vi "PobierzWiadomość.vi"(8 "error in":errorcluster, 9 "Ilość":string, 10 "Konto":T1, 11 "Typ wiadomości":string) -> (0 "error out":errorcluster, 3 "Wiadomość":string)   [LabVIEW 2021]
doc: "Return message in function of the message type\nAnd replace AMOUNT, NAME field in message"
uses:
  Konto.ctl
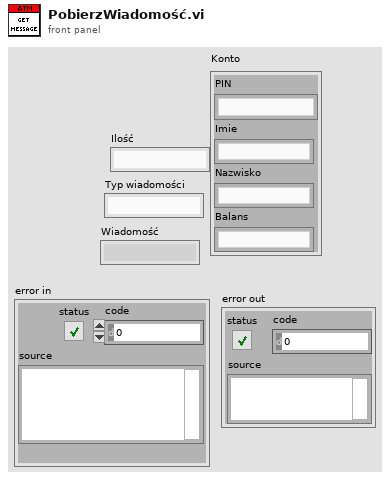
[diagram p1: front panel]
types:
  T1 = typedef "Konto.ctl" = cluster{"PIN":string, "Imie":string, "Nazwisko":string, "Balans":string}
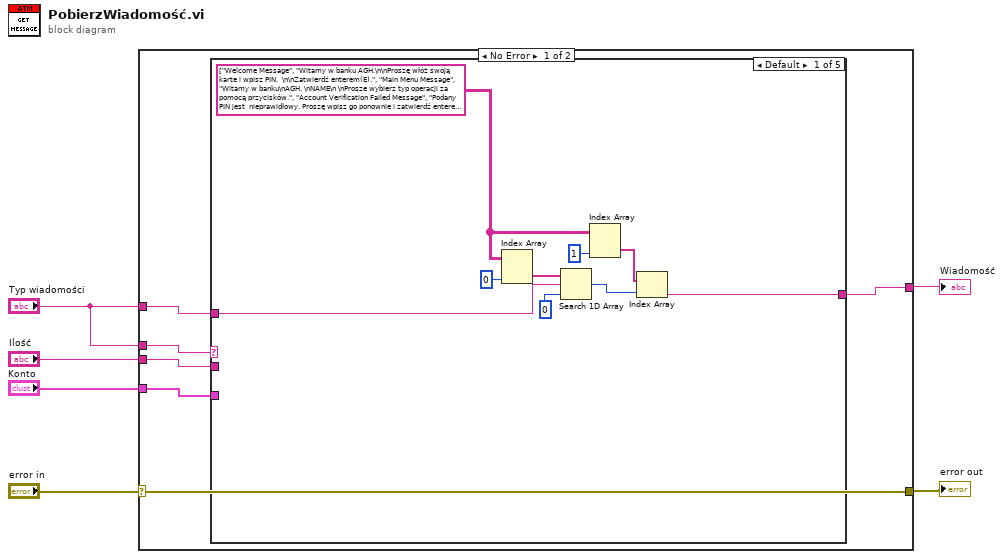
[diagram p0: block diagram]
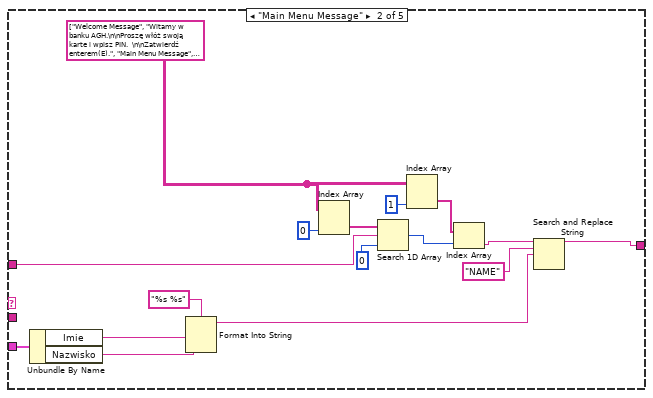
[diagram p2: hidden frame]
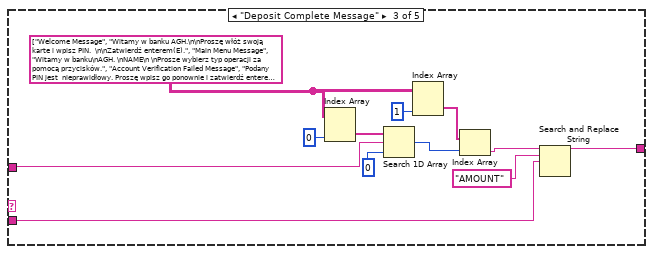
[diagram p3: hidden frame]
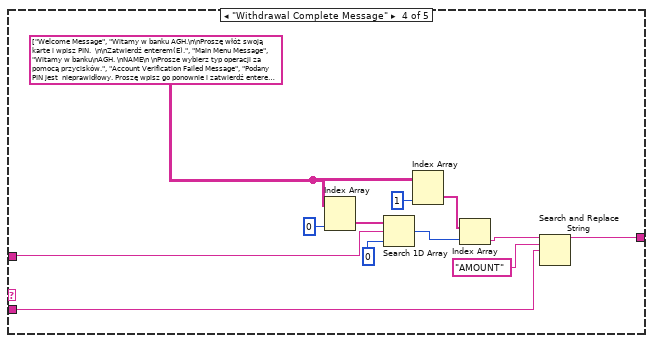
[diagram p4: hidden frame]
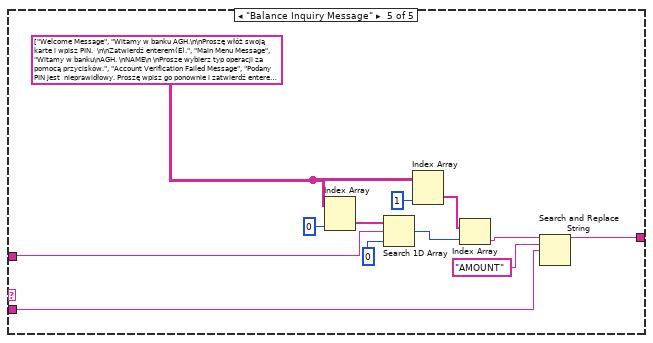
[diagram p5: hidden frame]
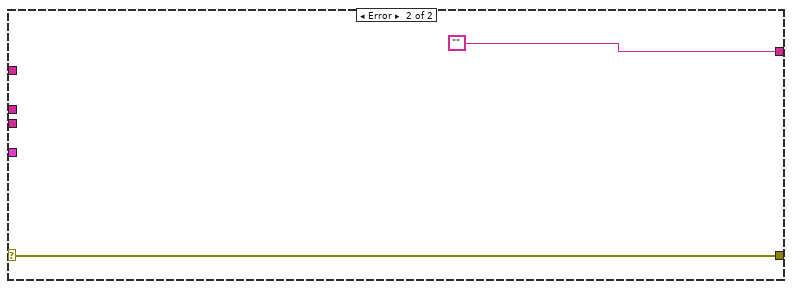
[diagram p6: hidden frame]
diagram:
  n1 = case shown="No Error" "error in" {
    selector: "error in" -> [w10 w75]
    tunnel: "Typ wiadomości" -> [w12 _]
    tunnel: [w11 ""] -> w6
    tunnel: [w10 w75] -> w4
    tunnel: "Typ wiadomości" -> [w9 _]
    tunnel: "Konto" -> [w8 _]
    tunnel: "Ilość" -> [w7 _]
    frame No Error {
      n2 = case shown="Default" w9 {
        tunnel: w12 -> [w14 w31 w40 w52 w64]
        tunnel: [w15 w23 w39 w51 w63] -> w11
        tunnel: w8 -> [_ w29 _ _ _]
        tunnel: w7 -> [_ _ w38 w50 w62]
        frame Default {
          w13 = string[][] [["Welcome Message", "Witamy w banku AGH.\n\nProszę włóż swoją karte i wpisz PIN.  \n\nZatwierdź enterem(E)."], ["Main Menu Message", "Witamy w banku\nAGH. \nNAME\n \nProsze wybierz typ operacji za pomocą przycisków."], ["Account Verification Failed Message", "Podany PIN jest  nieprawidłowy. Proszę wpisz go ponownie i zatwierdź enterem (E)."], ["Session Terminate Message", "Twoja sesja wygasła w związku z nieaktywnością.\nBy kontynuować zaloguj się ponownie. \n \nDo widzenia!"], ["Deposit Message", "Proszę wpisz kwotę jaką chcesz wpłacić i zatwierdź enterem (E)."], ["Deposit Complete Message", "AMOUNT zł\nWpłacono"], ["Withdrawal Message", "Proszę wpisz kwotę jaką chcesz wypłacić i zatwierdź enterem (E)."], ["Withdrawal Complete Message", "AMOUNT zł Wypłacono"], ["Withdrawal Failed Message", "Niewystarczająca ilość środków na koncie do przeprowadzenia transakcji. Spróbuj ponownie."], ["Balance Inquiry Message", "Twój stan konta wynosi: \nAMOUNT zł"]] ("Array")
          n3 = Index Array(array=w13, index (col)=0 ("disabled index (col)")) -> (element=w17:string[])  [unwired: 1 in]
          n4 = Search 1D Array(1D array=w17, element=w14, start index (0)=0) -> (index of element=w19:i32)
          n5 = Index Array(array=w13, index (col)=1 ("disabled index (col)")) -> (element=w21:string[])  [unwired: 1 in]
          n6 = Index Array(array=w21, index=w19) -> (element=w15:string)
        }
        frame "Main Menu Message" {
          w22 = string[][] [["Welcome Message", "Witamy w banku AGH.\n\nProszę włóż swoją karte i wpisz PIN.  \n\nZatwierdź enterem(E)."], ["Main Menu Message", "Witamy w banku AGH.\nNAME\n \nProszę wybrać rodzaj operacji\nprzy użyciu przycisków."], ["Account Verification Failed Message", "Podany PIN jest  nieprawidłowy. Proszę wpisz go ponownie i zatwierdź enterem (E)."], ["Session Terminate Message", "Twoja sesja wygasła w związku z nieaktywnością.\nBy kontynuować zaloguj się ponownie. \n \nDo widzenia! \ndue to inactivity or menu selection. \nPlease take your card \n \nGoodbye!"], ["Deposit Message", "Proszę wpisz kwotę jaką chcesz wpłacić i zatwierdź enterem (E)."], ["Deposit Complete Message", "AMOUNT zł\nWpłacono"], ["Withdrawal Message", "Proszę wpisz kwotę jaką chcesz wypłacić i zatwierdź enterem (E)."], ["Withdrawal Complete Message", "AMOUNT zł Wypłacono"], ["Withdrawal Failed Message", "Niewystarczająca ilość środków na koncie do przeprowadzenia transakcji. Spróbuj ponownie."], ["Balance Inquiry Message", "Twój stan konta wynosi: \n(Balance Amount from file) zł"]] ("Array")
          n7 = Unbundle By Name(w29) -> ("Imie"=w28:string, "Nazwisko"=w27:string)
          n8 = Format Into String(format string="%s %s", w28, w27) -> (resulting string=w24:string)  [unwired: 2 in, 1 out]
          n9 = Index Array(array=w22, index (col)=0 ("disabled index (col)")) -> (element=w36:string[])  [unwired: 1 in]
          n10 = Search 1D Array(1D array=w36, element=w31, start index (0)=0) -> (index of element=w34:i32)
          n11 = Index Array(array=w22, index (col)=1 ("disabled index (col)")) -> (element=w32:string[])  [unwired: 1 in]
          n12 = Index Array(array=w32, index=w34) -> (element=w26:string)
          n13 = Search and Replace String(input string=w26, search string="NAME", replace string=w24) -> (result string=w23:string)  [unwired: 5 in, 3 out]
        }
        frame "Deposit Complete Message" {
          w41 = string[][] [["Welcome Message", "Witamy w banku AGH.\n\nProszę włóż swoją karte i wpisz PIN.  \n\nZatwierdź enterem(E)."], ["Main Menu Message", "Witamy w banku\nAGH. \nNAME\n \nProsze wybierz typ operacji za pomocą przycisków."], ["Account Verification Failed Message", "Podany PIN jest  nieprawidłowy. Proszę wpisz go ponownie i zatwierdź enterem (E)."], ["Session Terminate Message", "Twoja sesja wygasła w związku z nieaktywnością.\nBy kontynuować zaloguj się ponownie. \n \nDo widzenia!"], ["Deposit Message", "Proszę wpisz kwotę jaką chcesz wpłacić i zatwierdź enterem (E)."], ["Deposit Complete Message", "AMOUNT zł\nWpłacono"], ["Withdrawal Message", "Proszę wpisz kwotę jaką chcesz wypłacić i zatwierdź enterem (E)."], ["Withdrawal Complete Message", "AMOUNT zł Wypłacono"], ["Withdrawal Failed Message", "Niewystarczająca ilość środków na koncie do przeprowadzenia transakcji. Spróbuj ponownie."], ["Balance Inquiry Message", "Twój stan konta wynosi: \n(Balance Amount from file) zł"]] ("Array")
          n14 = Index Array(array=w41, index (col)=0 ("disabled index (col)")) -> (element=w48:string[])  [unwired: 1 in]
          n15 = Search 1D Array(1D array=w48, element=w40, start index (0)=0) -> (index of element=w46:i32)
          n16 = Index Array(array=w41, index (col)=1 ("disabled index (col)")) -> (element=w44:string[])  [unwired: 1 in]
          n17 = Index Array(array=w44, index=w46) -> (element=w43:string)
          n18 = Search and Replace String(input string=w43, search string="AMOUNT", replace string=w38) -> (result string=w39:string)  [unwired: 5 in, 3 out]
        }
        frame "Withdrawal Complete Message" {
          w53 = string[][] [["Welcome Message", "Witamy w banku AGH.\n\nProszę włóż swoją karte i wpisz PIN.  \n\nZatwierdź enterem(E)."], ["Main Menu Message", "Witamy w banku\nAGH. \nNAME\n \nProsze wybierz typ operacji za pomocą przycisków."], ["Account Verification Failed Message", "Podany PIN jest  nieprawidłowy. Proszę wpisz go ponownie i zatwierdź enterem (E)."], ["Session Terminate Message", "Twoja sesja wygasła w związku z nieaktywnością.\nBy kontynuować zaloguj się ponownie. \n \nDo widzenia!"], ["Deposit Message", "Proszę wpisz kwotę jaką chcesz wpłacić i zatwierdź enterem (E)."], ["Deposit Complete Message", "AMOUNT zł\nWpłacono"], ["Withdrawal Message", "Proszę wpisz kwotę jaką chcesz wypłacić i zatwierdź enterem (E)."], ["Withdrawal Complete Message", "AMOUNT zł Wypłacono"], ["Withdrawal Failed Message", "Niewystarczająca ilość środków na koncie do przeprowadzenia transakcji. Spróbuj ponownie."], ["Balance Inquiry Message", "Twój stan konta wynosi: \n(Balance Amount from file) zł"]] ("Array")
          n19 = Index Array(array=w53, index (col)=0 ("disabled index (col)")) -> (element=w60:string[])  [unwired: 1 in]
          n20 = Search 1D Array(1D array=w60, element=w52, start index (0)=0) -> (index of element=w58:i32)
          n21 = Index Array(array=w53, index (col)=1 ("disabled index (col)")) -> (element=w56:string[])  [unwired: 1 in]
          n22 = Index Array(array=w56, index=w58) -> (element=w55:string)
          n23 = Search and Replace String(input string=w55, search string="AMOUNT", replace string=w50) -> (result string=w51:string)  [unwired: 5 in, 3 out]
        }
        frame "Balance Inquiry Message" {
          w65 = string[][] [["Welcome Message", "Witamy w banku AGH.\n\nProszę włóż swoją karte i wpisz PIN.  \n\nZatwierdź enterem(E)."], ["Main Menu Message", "Witamy w banku\nAGH. \nNAME\n \nProsze wybierz typ operacji za pomocą przycisków."], ["Account Verification Failed Message", "Podany PIN jest  nieprawidłowy. Proszę wpisz go ponownie i zatwierdź enterem (E)."], ["Session Terminate Message", "Twoja sesja wygasła w związku z nieaktywnością.\nBy kontynuować zaloguj się ponownie. \n \nDo widzenia!"], ["Deposit Message", "Proszę wpisz kwotę jaką chcesz wpłacić i zatwierdź enterem (E)."], ["Deposit Complete Message", "AMOUNT zł\nWpłacono"], ["Withdrawal Message", "Proszę wpisz kwotę jaką chcesz wypłacić i zatwierdź enterem (E)."], ["Withdrawal Complete Message", "AMOUNT zł Wypłacono"], ["Withdrawal Failed Message", "Niewystarczająca ilość środków na koncie do przeprowadzenia transakcji. Spróbuj ponownie."], ["Balance Inquiry Message", "Twój stan konta wynosi: \nAMOUNT zł"]] ("Array")
          n24 = Index Array(array=w65, index (col)=0 ("disabled index (col)")) -> (element=w72:string[])  [unwired: 1 in]
          n25 = Search 1D Array(1D array=w72, element=w64, start index (0)=0) -> (index of element=w70:i32)
          n26 = Index Array(array=w65, index (col)=1 ("disabled index (col)")) -> (element=w68:string[])  [unwired: 1 in]
          n27 = Index Array(array=w68, index=w70) -> (element=w67:string)
          n28 = Search and Replace String(input string=w67, search string="AMOUNT", replace string=w62) -> (result string=w63:string)  [unwired: 5 in, 3 out]
        }
      }
    }
    frame Error {
    }
  }
  "Wiadomość" <- w6
  "error out" <- w4
